vi "Close_Baxter.vi"(0 "error in":errorcluster, 3 "node":string) -> (1 "error out":errorcluster)   [LabVIEW 2012]
doc: "This will close all topics and disable Baxter."
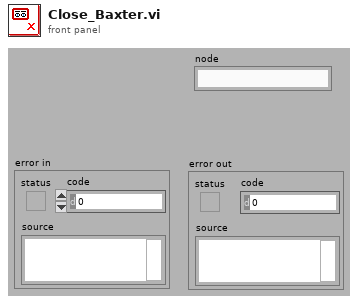
[diagram p1: front panel]
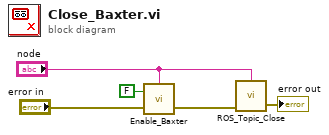
[diagram p0: block diagram]
diagram:
  n1 = call <userlib>:"Enable_Baxter.vi"("error in"="error in", "Enable?"=FALSE, "node"="node") -> ("error out"=w3:errorcluster)  [unwired: 1 in]
  n2 = call <userlib>:"ROS_Topic_Close.vi"("error in"=w3, "node"="node") -> ("error out"=→"error out":errorcluster)  [unwired: 2 in]
